vi "Test.vi"() -> ()   [LabVIEW 2014, in "Generic Power Analyzer.lvlib" / "Tektronix DMM4020.lvlib"]
uses:
  Tektronix DMM4020.lvlib
  Tektronix DMM4020.lvclass
  <vilib>/ActorFramework/Message Enqueuer/Message Enqueuer.lvclass/Message Enqueuer.ctl
  <vilib>/ActorFramework/Message Enqueuer/Enqueue.vi
  <vilib>/ActorFramework/Message Priority Queue/Priority Enqueue.vi
  <vilib>/ActorFramework/Stop Msg/Stop Msg.lvclass
  <vilib>/ActorFramework/Actor/Actor.lvclass
panel:
  out "error out":errorcluster
  in  "Stop Button":bool
  in  "VISA resource name":refnum<visa-resource-name>
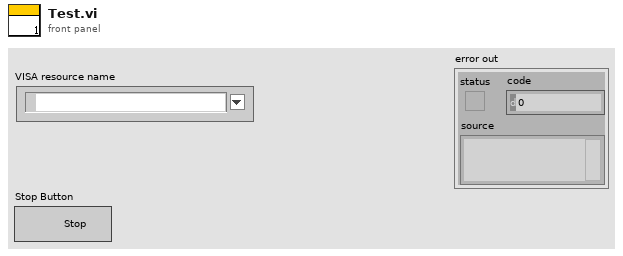
[diagram p1: front panel]
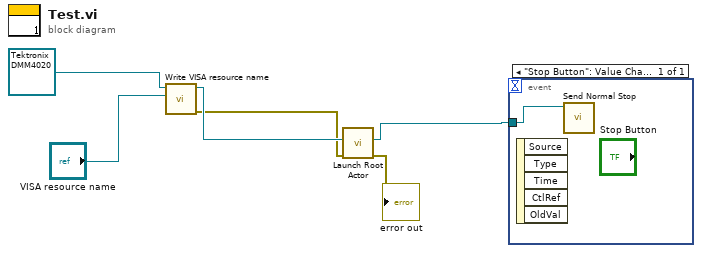
[diagram p0: block diagram]
diagram:
  n1 = call-dynamic "Write VISA resource name.vi"("VISA resource name"="VISA resource name", "Generic Instrument in"=refnum<class "Tektronix DMM4020.lvclass"> refnum ("Generic Power Analyzer.lvlib:Tektronix DMM4020.lvlib:Tektronix DMM4020.lvclass")) -> ("error out"=w1:errorcluster, "Generic Instrument out"=w4:refnum<class "Tektronix DMM4020.lvclass">)  [unwired: 8 in]
  n2 = call <vilib>:"Launch Root Actor.vi"("error in (no error)"=w1, "Actor"=w4) -> ("error out"=→"error out":errorcluster, "Actor's Enqueuer"=w3:refnum<class "Message Enqueuer.lvclass">)  [unwired: 8 in]
  n3 = event shown="[0] \"Stop Button\": Value Change" {
    selector: _ -> [_]
    dyn-events: _ -> [_]
    timeout: _ -> [_]
    tunnel: w3 -> [w7]
    event "Stop Button": Value Change {
      n4 = event-data() -> ()  [unwired: 1 in, 5 out]
      n5 = call <vilib>:"Send Normal Stop.vi"("Message Enqueuer"=w7) -> ()  [unwired: 10 in, 1 out]
    }
  }
